vi "DBSensorDataToArray.vi"(4 "begin":timestamp, 5 "plant":enum16{"B2G1", "B2G2"}(ring), 6 "load":bool, 7 "appended path":path, 8 "sensor":T1(ring), 9 "end":timestamp, 10 "shift reg out in":cluster{timestamp, dbl}[](array[cluster]), 11 "XYGraph in":refnum<vi>) -> (0 "error out":errorcluster, 3 "shift reg out":cluster{timestamp, dbl}[](array[cluster]))   [LabVIEW 2011]
uses:
  DBSqlSelectToArray(1DArrayClusterTimestampDouble).vi
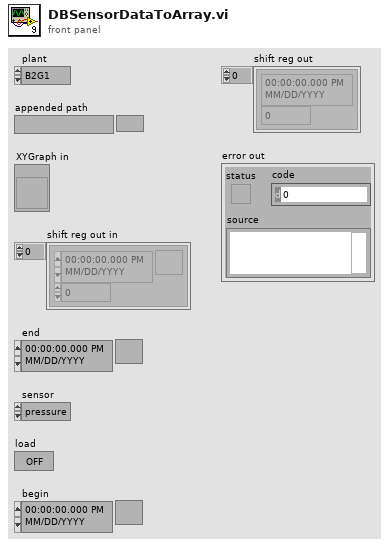
[diagram p1: front panel]
types:
  T1 = enum16{"pressure", "temperature 4", "temperature 5", "pH-value", "fill level 1", "fill level 2", "fill level 3"}
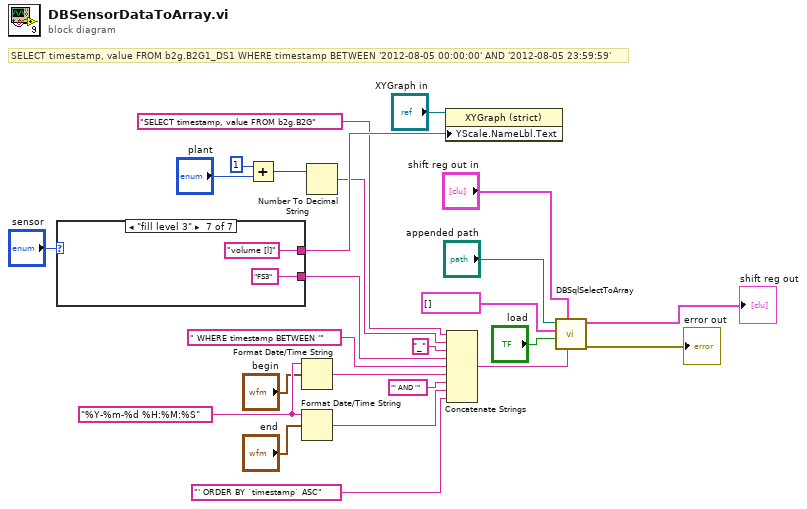
[diagram p0: block diagram]
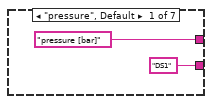
[diagram p2: hidden frame]
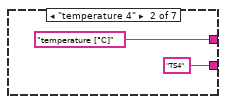
[diagram p3: hidden frame]
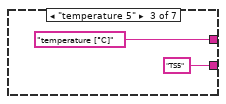
[diagram p4: hidden frame]
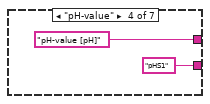
[diagram p5: hidden frame]
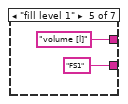
[diagram p6: hidden frame]
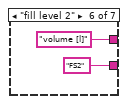
[diagram p7: hidden frame]
diagram:
  w22 = "%Y-%m-%d %H:%M:%S"
  # "SELECT timestamp, value FROM b2g.B2G1_DS1 WHERE timestamp BETWEEN '2012-08-05 00:00:00' AND '2012-08-05 23:59:59'"
  n1 = case shown="\"fill level 3\"" "sensor" {
    tunnel: ["DS1" "TS4" "TS5" "pHS1" "FS1" "FS2" "FS3"] -> w16
    tunnel: ["pressure [bar]" "temperature [°C]" "temperature [°C]" "pH-value [pH]" "volume [l]" "volume [l]" "volume [l]"] -> w25
    frame "pressure", Default {
    }
    frame "temperature 4" {
    }
    frame "temperature 5" {
    }
    frame "pH-value" {
    }
    frame "fill level 1" {
    }
    frame "fill level 2" {
    }
    frame "fill level 3" {
    }
  }
  n2 = Add(x=1, y="plant") -> (x+y=w13:i32)
  n3 = Format Date/Time String(time format string (%c)=w22, seconds (now)="begin") -> (date/time string=w19:string)  [unwired: 1 in]
  n4 = Format Date/Time String(time format string (%c)=w22, seconds (now)="end") -> (date/time string=w23:string)  [unwired: 1 in]
  n5 = Number To Decimal String(number=w13) -> (decimal integer string=w10:string)  [unwired: 1 in]
  n6 = property on="Property Node" class="XYGraph (strict)"(reference="XYGraph in", "YScale.NameLbl.Text"=w25) -> ()  [unwired: 1 in, 2 out]
  n7 = Concatenate Strings("SELECT timestamp, value FROM b2g.B2G", w10, "_", w16, " WHERE timestamp BETWEEN '", w19, "' AND '", w23, "' ORDER BY `timestamp` ASC") -> (w5:string)
  n8 = call-poly "DBSqlSelectToArray.vi"("String"=w5, "shift reg in"="shift reg out in", "enable"="load", "format"=cluster{timestamp, dbl}[] [] ("columns"), "connection information"="appended path") -> ("error out"=→"error out":errorcluster, "shift reg out"=→"shift reg out":cluster{timestamp, dbl}[])  [unwired: 5 in]
